vi "Get Main Config File Ref.vi"(8 "error in":errorcluster, 10 "Main VI Name":string, 11 "Main VI Directory":path) -> (0 "error out":errorcluster, 3 "Main Config File Refnum":T1)   [LabVIEW 2018]
doc: "Locates and opens a reference to an INI configuration file in the Main VI directory. This file is supposed to have the same name as the main top level VI, only with a .ini file extension.\n\n2007_11 Mike Ashe\nmichael.ashe@imaginatics.net\nCell: 860-961-0876"
uses:
  <vilib>/Utility/config.llb/Config Data RefNum.ctl
  <userlib>/_OpenG.lib/file/file.llb/Convert File Extension (Path)__ogtk.vi
  <vilib>/Utility/config.llb/NI_LVConfig.lvlib
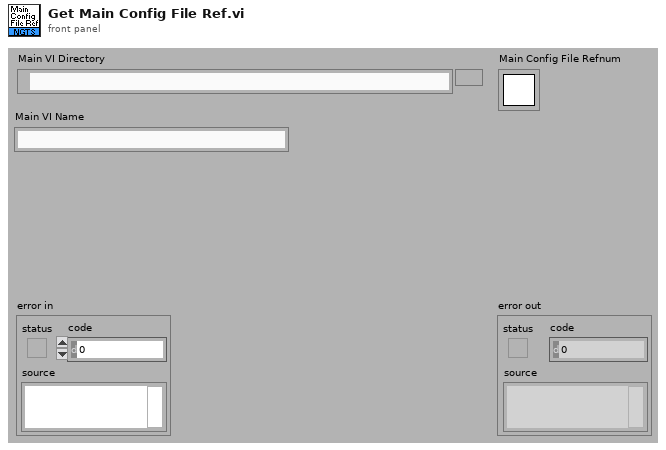
[diagram p1: front panel]
types:
  T1 = typedef "NI_LVConfig.lvlib/Config Data RefNum.ctl" = refnum<k1>
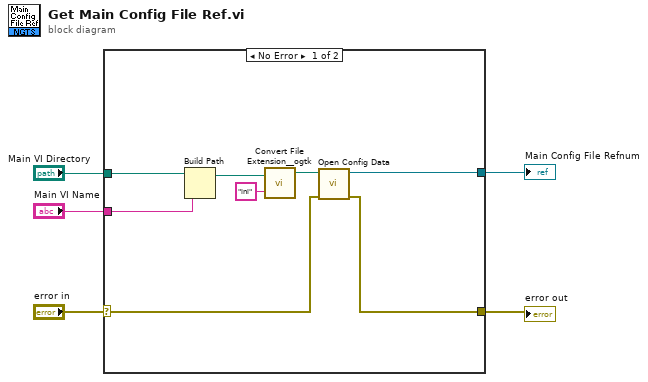
[diagram p0: block diagram]
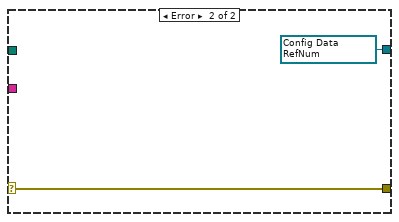
[diagram p2: hidden frame]
diagram:
  n1 = case shown="No Error" "error in" {
    selector: "error in" -> [w9 w15]
    tunnel: [w8 w15] -> w4
    tunnel: "Main VI Directory" -> [w13 _]
    tunnel: "Main VI Name" -> [w12 _]
    tunnel: [w6 w14] -> w1
    frame No Error {
      n2 = Build Path(base path=w13, name or relative path=w12) -> (appended path=w11:path)
      n3 = call-poly <userlib>:"Convert File Extension__ogtk.vi"("new ending (none)"="ini", "file name"=w11) -> ("new filename"=w7:path)  [unwired: 1 out]
      n4 = call <vilib>:"Open Config Data.vi"("error in (no error)"=w9, "configuration file path"=w7) -> ("error out"=w8:errorcluster, "refnum"=w6:T1)  [unwired: 7 in, 1 out]
    }
    frame Error {
      w14 = T1 refnum items=["config data"] ("refnum")
    }
  }
  "error out" <- w4
  "Main Config File Refnum" <- w1
